vi "App - FileSync Example.vi"() -> ()   [LabVIEW 2020]
uses:
  <userlib>/_NEVSTOP/Communicable State Machine(CSM)/addons/MassData-Parameter/Utility/Def-MassData Status Indicator(Vertical).ctl
  _fileSync_Support/Base/Def-FileSyncConfig.ctl
  CSM-FileSync.lvlib
  _fileSync_Support/Base/Protocol/Protocol.lvclass
  <userlib>/_NEVSTOP/Communicable State Machine(CSM)/Communicable State Machine.lvlib
  _fileSync_Support/FTP/FTPProtocol/FTPProtocol.lvclass
  D:/NEVSTOP-LAB-Development/CSMF/CSM-ModSets-FileSync/src/_fileSync_Support/Base/Protocol/Protocol.lvclass
panel:
  in  "MassData Status":T1 {"r" scale=1.0..50000000.0 scale format="%#_6p"; "w" scale=1.0..50000000.0 scale format="%#_6p"}
  in  "stop":bool
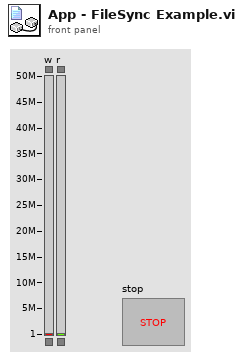
[diagram p1: front panel]
types:
  T1 = typedef "Def-MassData Status Indicator(Vertical).ctl" = cluster{"w":cluster{dbl, dbl}, "r":cluster{dbl, dbl}}
  T2 = typedef "FileSync -- Base.lvlib/Protocol.lvclass/Def-FileSyncConfig.ctl" = cluster{"MonitoringFolder":path, "BackupFolder":path, "autostart":bool, "Backup":bool}
  T3 = cluster{"address":string, "remote port":u16, "userName":string, "passWord":string, "RootDir":string}
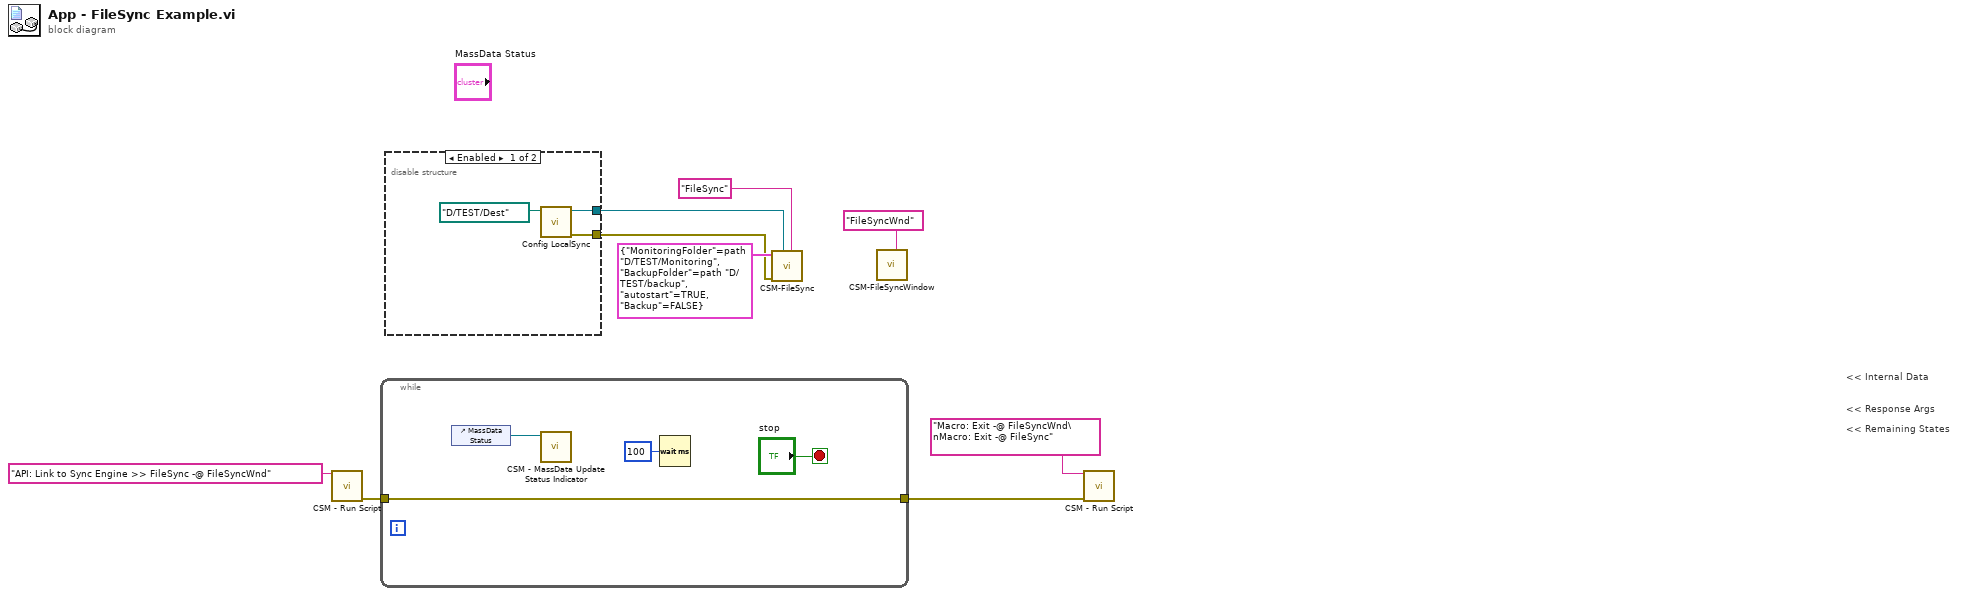
[diagram p0: block diagram]
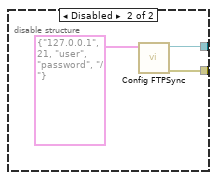
[diagram p2: hidden frame]
diagram:
  # "<< Internal Data"
  # "<< Response Args"
  # "<< Remaining States"
  n1 = call <userlib>:"CSM - Run Script.vi"("CSM Scripts"="API: Link to Sync Engine >> FileSync -@ FileSyncWnd") -> ("error out"=w4:errorcluster)  [unwired: 12 in, 2 out]
  n2 = while {
    tunnel: w4 -> [w10]
    tunnel: [w10] -> w1
    stop <- "stop" stop-if-true
    n3 = control-ref of="MassData Status"() -> (w11:refnum<vi>)
    n4 = call <userlib>:"CSM - MassData Update Status Indicator.vi"("MassData Status Indicator"=w11) -> ()  [unwired: 10 in, 1 out]
    n5 = Wait (ms)(milliseconds to wait=u32 100) -> ()  [unwired: 1 out]
  }
  n6 = disable-structure shown="Enabled" {
    disable-tunnel: [w16 w19] -> w8
    disable-tunnel: [w14 w17] -> w5
    frame Enabled {
      n7 = call "Config LocalSync.vi"("Dir"=path "D:/TEST/Dest") -> ("error out"=w14:errorcluster, "Protocol out"=w16:refnum<class "Protocol.lvclass">)  [unwired: 9 in]
    }
    frame Disabled {
      n8 = call "Config FTPSync.vi"("Cluster"=T3 {"address"="127.0.0.1", "remote port"=21, "userName"="user", "passWord"="password", "RootDir"="/"}) -> ("error out"=w17:errorcluster, "FTPProtocol out"=w19:refnum<class "FTPProtocol.lvclass">)  [unwired: 9 in]
    }
  }
  n9 = call "CSM-FileSync.vi"("Name(FileSync)"="FileSync", "Protocol.lvclass"=w8, "error in"=w5, "FileSync Configuration"=T2 {"MonitoringFolder"=path "D:/TEST/Monitoring", "BackupFolder"=path "D:/TEST/backup", "autostart"=TRUE, "Backup"=FALSE}) -> ()  [unwired: 7 in, 1 out]
  n10 = call "CSM-FileSyncWindow.vi"("Name(FileSync)"="FileSyncWnd") -> ()  [unwired: 10 in, 1 out]
  n11 = call <userlib>:"CSM - Run Script.vi"("CSM Scripts"="Macro: Exit -@ FileSyncWnd\nMacro: Exit -@ FileSync", "error in (no error)"=w1) -> ()  [unwired: 11 in, 3 out]
